vi "Write ColumnHeadersVisible.vi"(8 "error in (no error)":errorcluster, 10 "ColumnHeadersVisible":bool=TRUE, 11 "DataGridView in":refnum<class "DataGridView.lvclass">) -> (0 "error out":errorcluster, 3 "DataGridView out":refnum<class "DataGridView.lvclass">)   [LabVIEW 2014, in "DataGridView.lvclass"]
uses:
  DataGridView.lvclass
  DataGridView.lvclass/DataGridView.ctl
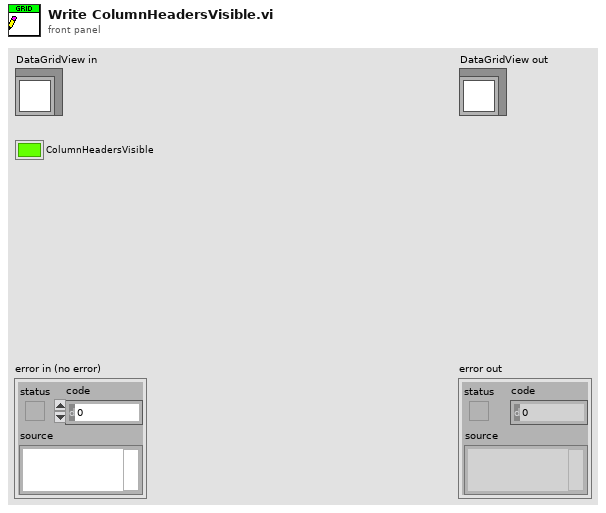
[diagram p1: front panel]
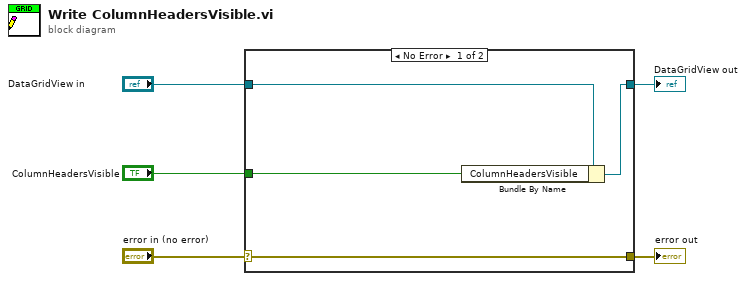
[diagram p0: block diagram]
diagram:
  n1 = case shown="No Error" "error in (no error)" {
    selector: "error in (no error)" -> [w9 w10]
    tunnel: [w9 w10] -> w4
    tunnel: [w7 w11] -> w2
    tunnel: "DataGridView in" -> [w8 w11]
    tunnel: "ColumnHeadersVisible" -> [w6 _]
    frame No Error {
      n2 = Bundle By Name(cluster=w8, "ColumnHeadersVisible"=w6) -> (w7:refnum<class "DataGridView.lvclass">)
    }
    frame Error {
    }
  }
  "error out" <- w4
  "DataGridView out" <- w2
